vi "passIfEqual.vi"(6 "delta (optional)":variant, 7 "custom report message (\"\")":string, 8 "error in (no error)":errorcluster, 9 "y":variant, 10 "x":variant, 11 "TestCase in":refnum<class "TestCase.lvclass">) -> (0 "error out":errorcluster, 3 "TestCase out":refnum<class "TestCase.lvclass">)   [LabVIEW 2013, in "TestCase.lvclass"]
doc: "Pass test if 'x' = 'y'. 'delta (optional)' if specified must be a numeric format and forces 'x', 'y' to be numeric. If 'delta' is not specified, x,y can be any variant data."
uses:
  TestCase.lvclass
  TestCase.lvclass/TestCase.ctl
  Libraries/VITesterUtilities.lvlib
panel:
  # "JKI VI Tester for LabVIEW\nhttp://jkisoft.com/vi-tester\nCopyright (C) 2007-2009, JKI <info@jkisoft.com>\nALL RIGHTS RESERVED"
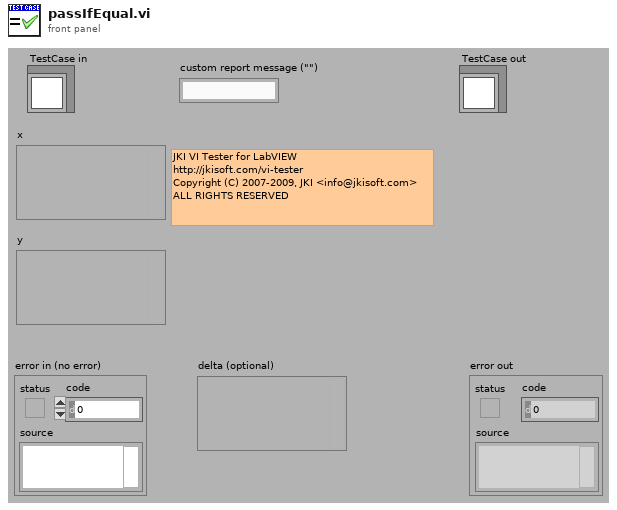
[diagram p1: front panel]
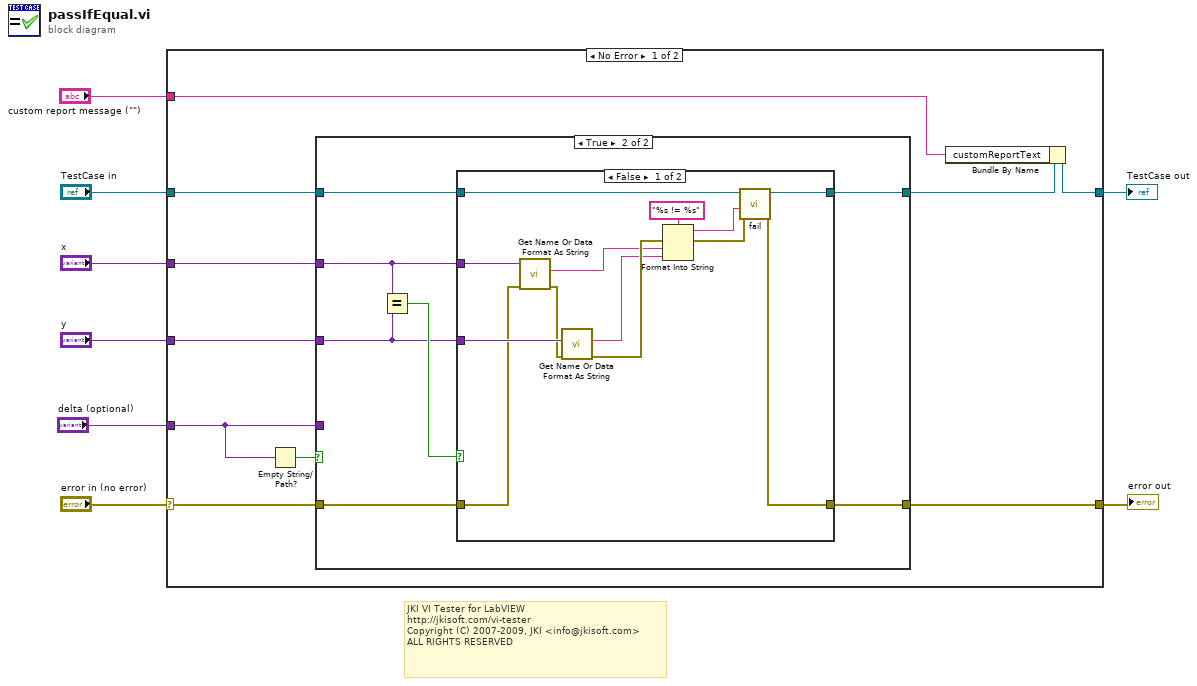
[diagram p0: block diagram]
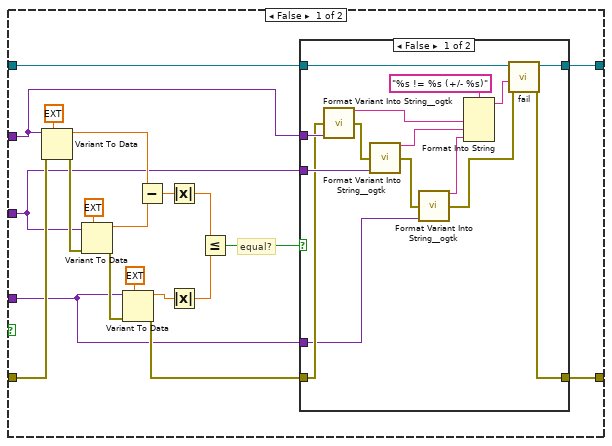
[diagram p2: hidden frame]
diagram:
  # "JKI VI Tester for LabVIEW\nhttp://jkisoft.com/vi-tester\nCopyright (C) 2007-2009, JKI <info@jkisoft.com>\nALL RIGHTS RESERVED"
  n1 = case shown="No Error" "error in (no error)" {
    selector: "error in (no error)" -> [w15 w79]
    tunnel: [w14 w79] -> w7
    tunnel: [w10 w78] -> w5
    tunnel: "TestCase in" -> [w12 w78]
    tunnel: "delta (optional)" -> [w13 _]
    tunnel: "x" -> [w18 _]
    tunnel: "y" -> [w17 _]
    tunnel: "custom report message (\"\")" -> [w9 _]
    frame No Error {
      n2 = Empty String/Path?(string/path=w13) -> (empty?=w16:bool)
      n3 = case shown="True" w16 {
        tunnel: w18 -> [w21 w57]
        tunnel: w17 -> [w20 w56]
        tunnel: w15 -> [w35 w61]
        tunnel: [w24 w60] -> w14
        tunnel: w13 -> [w19 _]
        tunnel: w12 -> [w23 w59]
        tunnel: [w22 w58] -> w11
        frame False {
          # "equal?"
          n4 = Variant To Data(error in=w35, type=ext 0.0, Variant=w21) -> (data=w32:ext, error out=w36:errorcluster)
          n5 = Variant To Data(error in=w36, type=ext 0.0, Variant=w20) -> (data=w31:ext, error out=w33:errorcluster)
          n6 = Variant To Data(error in=w33, type=ext 0.0, Variant=w19) -> (data=w29:ext, error out=w25:errorcluster)
          n7 = Subtract(x=w32, y=w31) -> (x-y=w30:ext)
          n8 = Absolute Value(x=w30) -> (abs(x)=w28:ext)
          n9 = Absolute Value(x=w29) -> (abs(x)=w27:ext)
          n10 = Less Or Equal?(x=w28, y=w27) -> (x <= y?=w26:bool)
          n11 = case shown="False" w26 {
            tunnel: [w53 w55] -> w24
            tunnel: w25 -> [w47 w55]
            tunnel: w23 -> [w52 w54]
            tunnel: [w51 w54] -> w22
            tunnel: w21 -> [w50 _]
            tunnel: w20 -> [w48 _]
            tunnel: w19 -> [w42 _]
            frame False {
              n12 = call <userlib>:"Format Variant Into String__ogtk.vi"("error in (no error)"=w47, "Variant"=w50) -> ("Output String"=w45:string, "error out"=w49:errorcluster)  [unwired: 12 in]
              n13 = call <userlib>:"Format Variant Into String__ogtk.vi"("error in (no error)"=w49, "Variant"=w48) -> ("Output String"=w46:string, "error out"=w40:errorcluster)  [unwired: 12 in]
              n14 = call <userlib>:"Format Variant Into String__ogtk.vi"("error in (no error)"=w40, "Variant"=w42) -> ("Output String"=w41:string, "error out"=w39:errorcluster)  [unwired: 12 in]
              n15 = Format Into String(format string="%s != %s (+/- %s)", w45, w46, w41) -> (resulting string=w43:string)  [unwired: 2 in, 1 out]
              n16 = call-dynamic "fail.vi"("error in (no error)"=w39, "message (\"\")"=w43, "TestCase in"=w52) -> ("error out"=w53:errorcluster, "TestCase out"=w51:refnum<class "TestCase.lvclass">)  [unwired: 7 in]
            }
            frame True {
            }
          }
        }
        frame True {
          n17 = Equal?(x=w57, y=w56) -> (x = y?=w62:bool)
          n18 = case shown="False" w62 {
            tunnel: w61 -> [w67 w76]
            tunnel: [w73 w76] -> w60
            tunnel: w59 -> [w72 w77]
            tunnel: [w71 w77] -> w58
            tunnel: w57 -> [w69 _]
            tunnel: w56 -> [w68 _]
            frame False {
              n19 = call "Get Name Or Data Format As String.vi"("error in (no error)"=w67, "Data"=w69) -> ("error out"=w66:errorcluster, "Data Value OR Name"=w63:string)  [unwired: 8 in]
              n20 = call "Get Name Or Data Format As String.vi"("error in (no error)"=w66, "Data"=w68) -> ("error out"=w65:errorcluster, "Data Value OR Name"=w64:string)  [unwired: 8 in]
              n21 = Format Into String(format string="%s != %s", error in=w65, w63, w64) -> (resulting string=w74:string, error out=w70:errorcluster)  [unwired: 1 in]
              n22 = call-dynamic "fail.vi"("error in (no error)"=w70, "message (\"\")"=w74, "TestCase in"=w72) -> ("error out"=w73:errorcluster, "TestCase out"=w71:refnum<class "TestCase.lvclass">)  [unwired: 7 in]
            }
            frame True {
            }
          }
        }
      }
      n23 = Bundle By Name(cluster=w11, "customReportText"=w9) -> (w10:refnum<class "TestCase.lvclass">)
    }
    frame Error {
    }
  }
  "error out" <- w7
  "TestCase out" <- w5
